vi "GetSpectrumParameterInfo.vi"(8 "error in":errorcluster, 10 "Parameter Name":string, 11 "connection ID in":refnum<k5>) -> (0 "error out":errorcluster, 1 "Error Info":T1, 2 "Spectrum Parameter Info":T2, 3 "connection ID out":refnum<k5>, 4 "Log String":string, 5 "OK":bool)   [LabVIEW 2015, in "ProdigyRemoteControl.lvlib"]
uses:
  ProdigyRemoteControl.lvlib
  DEFINITIONS/DEF_SpectrumParaInfo.ctl
  DEFINITIONS/DEF_RcError.ctl
  DEFINITIONS/DEF_RcCmd.ctl
  <vilib>/regexp/Match Regular Expression.xnode
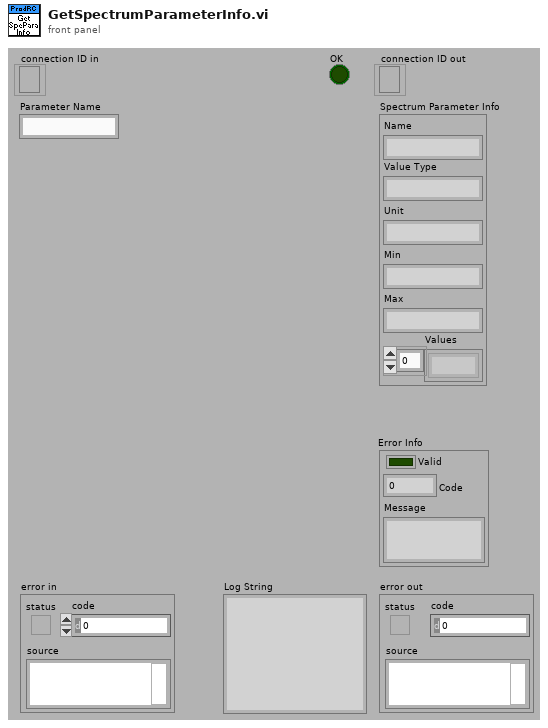
[diagram p1: front panel]
types:
  T1 = typedef "ProdigyRemoteControl.lvlib/DEF_RcError.ctl" = cluster{"Valid":bool, "Code":u16, "Message":string}
  T2 = typedef "ProdigyRemoteControl.lvlib/DEF_SpectrumParaInfo.ctl" = cluster{"Name":string, "Value Type":string, "Unit":string, "Min":string, "Max":string, "Values":string[]}
  T3 = typedef "ProdigyRemoteControl.lvlib/DEF_RcCmd.ctl" = string
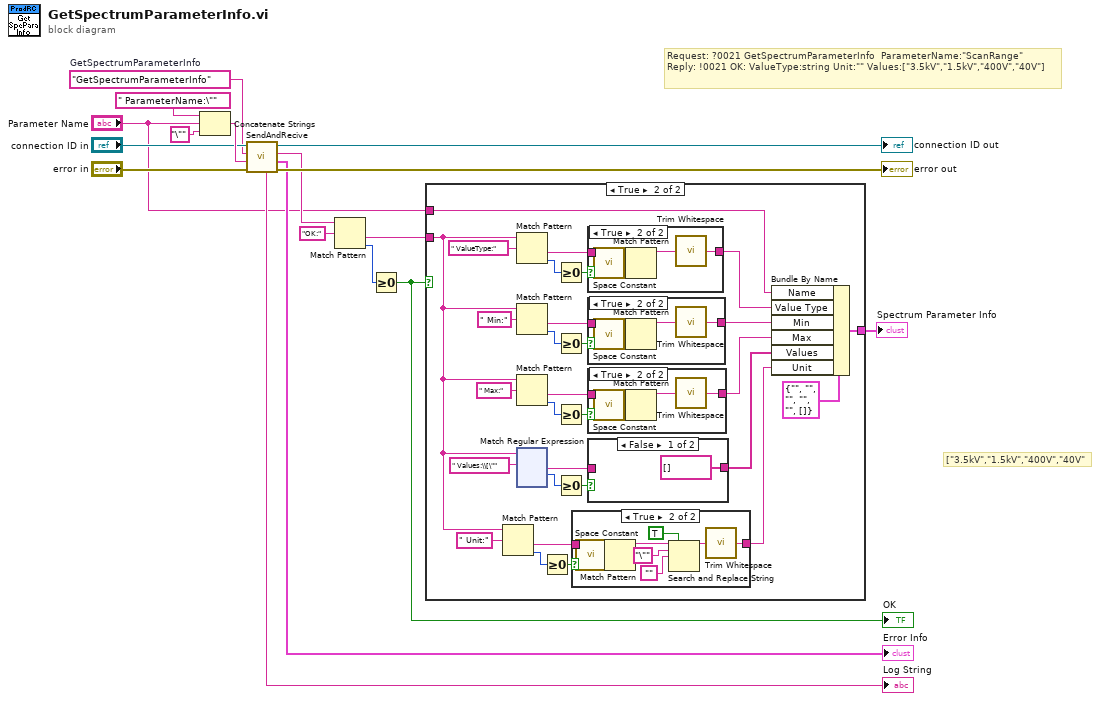
[diagram p0: block diagram]
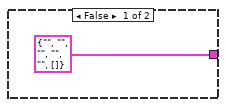
[diagram p2: hidden frame]
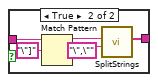
[diagram p3: hidden frame]
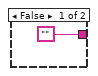
[diagram p4: hidden frame]
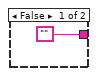
[diagram p5: hidden frame]
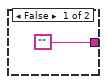
[diagram p6: hidden frame]
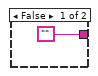
[diagram p7: hidden frame]
diagram:
  w1 = T3 "GetSpectrumParameterInfo"  # GetSpectrumParameterInfo
  # "Request: ?0021 GetSpectrumParameterInfo  ParameterName:\"ScanRange\"\nReply: !0021 OK: ValueType:string Unit:\"\" Values:[\"3.5kV\",\"1.5kV\",\"400V\",\"40V\"]"
  # "[\"3.5kV\",\"1.5kV\",\"400V\",\"40V\""
  n1 = Concatenate Strings(" ParameterName:\"", "Parameter Name", "\"" ("string")) -> (w17:string)
  n2 = call "SendAndRecive.vi"("error in"="error in", "Parameters"=w17, "Command"=w1, "connection ID in"="connection ID in") -> ("error out"=→"error out":errorcluster, "Error Info"=→"Error Info":T1, "Answer"=w8:string, "connection ID out"=→"connection ID out":refnum<k5>, "Log String"=→"Log String":string)  [unwired: 3 in]
  n3 = Match Pattern(string=w8, regular expression="OK:") -> (after substring=w4:string, offset past match=w6:i32)  [unwired: 1 in, 2 out]
  n4 = Greater Or Equal To 0?(x=w6) -> (x >= 0?=w5:bool)
  "OK" <- w5
  n5 = case shown="True" w5 {
    tunnel: w4 -> [_ w20]
    tunnel: "Parameter Name" -> [_ w27]
    tunnel: [T2 {"Name"="", "Value Type"="", "Unit"="", "Min"="", "Max"="", "Values"=[]} ("DEF_ParameterInfo") w22] -> w2
    frame False {
    }
    frame True {
      n6 = Match Pattern(string=w20, regular expression=" Unit:") -> (after substring=w42:string, offset past match=w43:i32)  [unwired: 1 in, 2 out]
      n7 = Match Pattern(string=w20, regular expression=" ValueType:") -> (after substring=w45:string, offset past match=w44:i32)  [unwired: 1 in, 2 out]
      n8 = Match Pattern(string=w20, regular expression=" Min:") -> (after substring=w37:string, offset past match=w36:i32)  [unwired: 1 in, 2 out]
      n9 = Match Pattern(string=w20, regular expression=" Max:") -> (after substring=w34:string, offset past match=w35:i32)  [unwired: 1 in, 2 out]
      n10 = xnode "Match Regular Expression"("input string"=w20, "regular expression"=" Values:\\[\"") -> ("after match"=w29:string, "offset past match"=w19:i32)  [unwired: 4 in, 3 out]
      n11 = Greater Or Equal To 0?(x=w43) -> (x >= 0?=w40:bool)
      n12 = Greater Or Equal To 0?(x=w44) -> (x >= 0?=w47:bool)
      n13 = Greater Or Equal To 0?(x=w36) -> (x >= 0?=w39:bool)
      n14 = Greater Or Equal To 0?(x=w35) -> (x >= 0?=w32:bool)
      n15 = Greater Or Equal To 0?(x=w19) -> (x >= 0?=w31:bool)
      n16 = case shown="True" w40 {
        tunnel: w42 -> [_ w183]
        tunnel: ["" w176] -> w21
        frame False {
        }
        frame True {
          n17 = call <vilib>:"Space Constant.vi"() -> ("String"=w182:string)
          n18 = Match Pattern(string=w183, regular expression=w182) -> (before substring=w180:string)  [unwired: 1 in, 3 out]
          n19 = Search and Replace String(replace all?=TRUE ("replace all? (F)"), input string=w180, search string="\"", replace string="") -> (result string=w181:string)  [unwired: 4 in, 3 out]
          n20 = call <vilib>:"Trim Whitespace.vi"("string"=w181) -> ("trimmed string"=w176:string)  [unwired: 1 in]
        }
      }
      n21 = case shown="True" w47 {
        tunnel: w45 -> [_ w188]
        tunnel: ["" w186] -> w26
        frame False {
        }
        frame True {
          n22 = call <vilib>:"Space Constant.vi"() -> ("String"=w187:string)
          n23 = Match Pattern(string=w188, regular expression=w187) -> (before substring=w185:string)  [unwired: 1 in, 3 out]
          n24 = call <vilib>:"Trim Whitespace.vi"("string"=w185) -> ("trimmed string"=w186:string)  [unwired: 1 in]
        }
      }
      n25 = case shown="True" w39 {
        tunnel: w37 -> [_ w174]
        tunnel: ["" w172] -> w25
        frame False {
        }
        frame True {
          n26 = call <vilib>:"Space Constant.vi"() -> ("String"=w173:string)
          n27 = Match Pattern(string=w174, regular expression=w173) -> (before substring=w171:string)  [unwired: 1 in, 3 out]
          n28 = call <vilib>:"Trim Whitespace.vi"("string"=w171) -> ("trimmed string"=w172:string)  [unwired: 1 in]
        }
      }
      n29 = case shown="True" w32 {
        tunnel: w34 -> [_ w169]
        tunnel: ["" w167] -> w24
        frame False {
        }
        frame True {
          n30 = call <vilib>:"Space Constant.vi"() -> ("String"=w168:string)
          n31 = Match Pattern(string=w169, regular expression=w168) -> (before substring=w166:string)  [unwired: 1 in, 3 out]
          n32 = call <vilib>:"Trim Whitespace.vi"("string"=w166) -> ("trimmed string"=w167:string)  [unwired: 1 in]
        }
      }
      n33 = case shown="False" w31 {
        tunnel: w29 -> [_ w164]
        tunnel: [string[] [] ("Strings") w161] -> w23
        frame False {
        }
        frame True {
          n34 = Match Pattern(string=w164, regular expression="\"]") -> (before substring=w162:string)  [unwired: 1 in, 3 out]
          n35 = call "SplitStrings.vi"("Delimiter String"="\",\"", "Input String"=w162) -> ("Strings"=w161:string[])  [unwired: 9 in]
        }
      }
      n36 = Bundle By Name(cluster=T2 {"Name"="", "Value Type"="", "Unit"="", "Min"="", "Max"="", "Values"=[]} ("DEF_ParameterInfo"), "Name"=w27, "Value Type"=w26, "Min"=w25, "Max"=w24, "Values"=w23, "Unit"=w21) -> (w22:T2)
    }
  }
  "Spectrum Parameter Info" <- w2
